vi "Create Evaluations.vi"(8 "error in (no error)":errorcluster, 11 "IEvaluation in":refnum<class "TDSCDMA_ACP.lvclass">) -> (0 "error out":errorcluster, 2 "Evaluations Out":T1[](array[typedef]) {"Low Limit" format="%#_13g"; "SI Scaling" items=["femto"=-15, "pico"=-12, "nano"=-9, "micro"=-6, "milli"=-3, "percent"=-2, ""=0, "kilo"=3, "mega"=6, "giga"=9, "tera"=12]}, 3 "IEvaluation out":refnum<class "TDSCDMA_ACP.lvclass">)   [LabVIEW 2016, in "SeqAuto Evaluations.lvlib" / "TDSCDMA_ACP.lvclass"]
uses:
  TDSCDMA_ACP.lvclass
  C:/projects/STS/Common/Sequence Automation/Plugins/SeqAuto IEvaluation.lvlibp/SeqAuto IEvaluation.lvclass
  Plugins/TestStand API Tools (TSAT).lvlibp/Evaluation Actions/Includes/Controls/TSAT Evaluation.ctl
  Plugins/TestStand API Tools (TSAT).lvlibp/Evaluation Actions/Includes/Controls/TSAT Eval SI Unit Scaling.ctl
  Plugins/TestStand API Tools (TSAT).lvlibp/Evaluation Actions/Includes/Controls/TSAT Evaluation Type.ctl
  TDSCDMA_ACP.lvclass/TDSCDMA_ACP.ctl
  Plugins/SeqAuto IEvaluation.lvlibp/Read Measurement Name.vi
  Plugins/TestStand API Tools (TSAT).lvlibp/Evaluation Actions/TSAT Evaluation Actions.lvlib
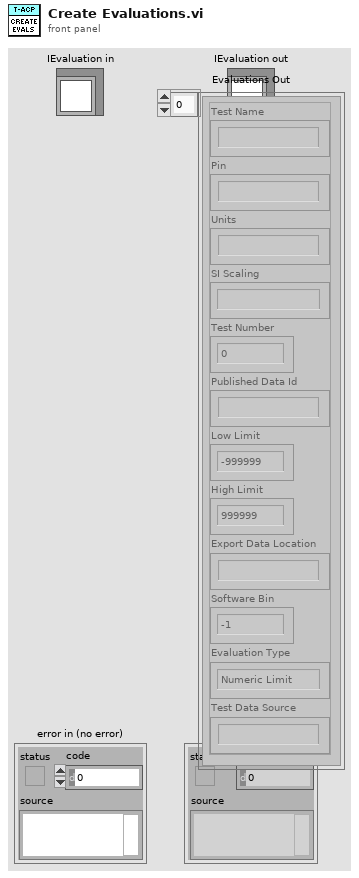
[diagram p1: front panel]
types:
  T1 = typedef "TestStand API Tools (TSAT).lvlibp/TSAT Evaluation Actions.lvlib/TSAT Evaluation.ctl" = cluster{"Test Name":string, "Pin":string, "Units":string, "SI Scaling":T2, "Test Number":i32, "Published Data Id":string, "Low Limit":dbl, "High Limit":dbl, "Export Data Location":string, "Software Bin":i64, "Evaluation Type":T3, "Test Data Source":string}
  T2 = typedef "TestStand API Tools (TSAT).lvlibp/TSAT Evaluation Actions.lvlib/TSAT Eval SI Unit Scaling.ctl" = i16
  T3 = typedef "TestStand API Tools (TSAT).lvlibp/TSAT Evaluation Actions.lvlib/TSAT Evaluation Type.ctl" = enum16{"Numeric Limit", "Pass/Fail", "None"}
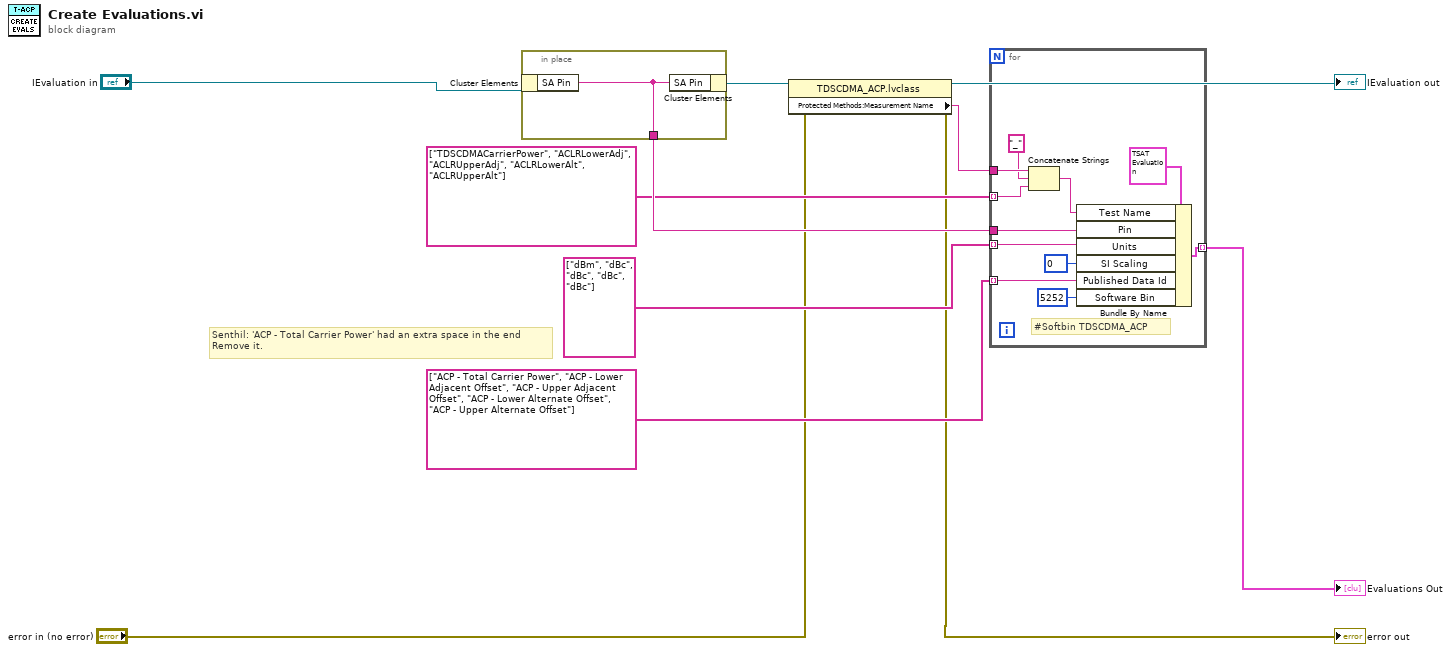
[diagram p0: block diagram]
diagram:
  # "Senthil: 'ACP - Total Carrier Power' had an extra space in the end\nRemove it."
  n1 = in-place {
    in-place-border: [w12] -> w10
    n2 = in-place-cluster #1("IEvaluation in") -> ("SA Pin"=w12:string)
    n3 = in-place-cluster #1("SA Pin"=w12) -> (w11:refnum<class "TDSCDMA_ACP.lvclass">)
  }
  n4 = property class="TDSCDMA_ACP.lvclass"(reference=w11, error in="error in (no error)") -> (reference out=→"IEvaluation out":refnum<class "TDSCDMA_ACP.lvclass">, error out=→"error out":errorcluster, "Protected Methods:Measurement Name"=w7:string)
  n5 = for {
    tunnel: w10 -> [w22]
    tunnel: string[] ["dBm", "dBc", "dBc", "dBc", "dBc"] -> [w21] mode=indexing
    tunnel: string[] ["ACP - Total Carrier Power", "ACP - Lower Adjacent Offset", "ACP - Upper Adjacent Offset", "ACP - Lower Alternate Offset", "ACP - Upper Alternate Offset"] -> [w20] mode=indexing
    tunnel: [w19] -> w3 mode=indexing
    tunnel: w7 -> [w17]
    tunnel: string[] ["TDSCDMACarrierPower", "ACLRLowerAdj", "ACLRUpperAdj", "ACLRLowerAlt", "ACLRUpperAlt"] -> [w16] mode=indexing
    w14 = T2 0 items=["femto"=-15, "pico"=-12, "nano"=-9, "micro"=-6, "milli"=-3, "percent"=-2, ""=0, "kilo"=3, "mega"=6, "giga"=9, "tera"=12] ("SI Scaling")
    # "#Softbin TDSCDMA_ACP"
    n6 = Concatenate Strings(w17, "_" ("string"), w16) -> (w18:string)
    n7 = Bundle By Name(cluster=T1 {"Test Name"="", "Pin"="", "Units"="", "SI Scaling"=0, "Test Number"=0, "Published Data Id"="", "Low Limit"=-999999.0, "High Limit"=999999.0, "Export Data Location"="", "Software Bin"=-1, "Evaluation Type"=enum."Numeric Limit", "Test Data Source"=""} ("Evaluation"), "Test Name"=w18, "Pin"=w22, "Units"=w21, "SI Scaling"=w14, "Published Data Id"=w20, "Software Bin"=i64 5252) -> (w19:T1)
  }
  "Evaluations Out" <- w3
